vi "makeChangelogSVN.vi"(9 "end":string(combo) caption="endTagOrHash", 10 "start":string(combo) caption="startTagOrHash", 11 "VI Path":path) -> (1 "Changelog":string)   [LabVIEW 2022 SP3]
uses:
  d1585840-c92d-4c4b-9acf-e53ee60be502.vi
  <vilib>/Comparison/Less/Less Functor/Less Functor.lvclass
panel:
  in  "Tab Control":enum32{"changelog", "subVIs", "svn log"}(tab)
  out "subVIs":string[](array[string])
  out "standard output":string
  out "commandline":string="2.years"
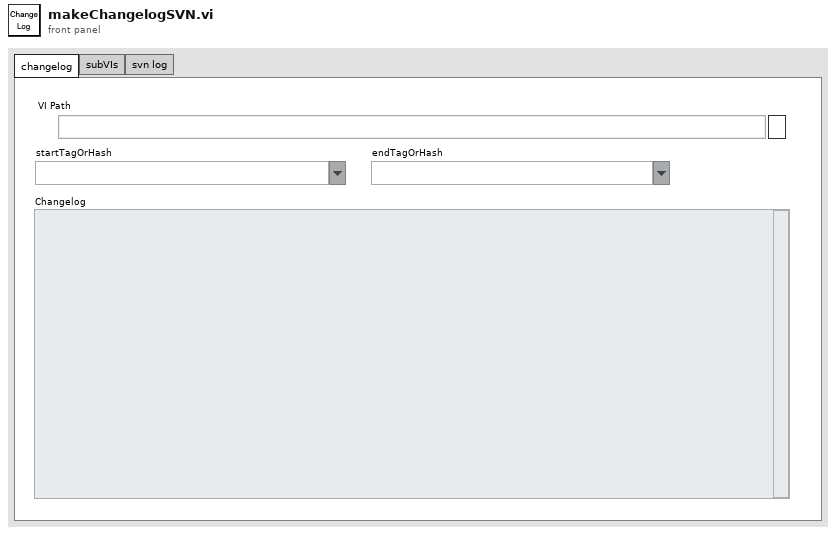
[diagram p1: front panel]
types:
  T1 = enum8{"Only include commented out diagrams if diagram already loaded", "Never include commented out diagrams", "Always include commented out diagrams"}
  T2 = enum8{"No dynamic dispatch VIs", "Include nearest implementation", "Include all overrides"}
  T3 = enum8{"Include the clone VI", "Include the original reentrant VI instead of the clone VI", "Include both the original reentrant VI and the clone VI"}
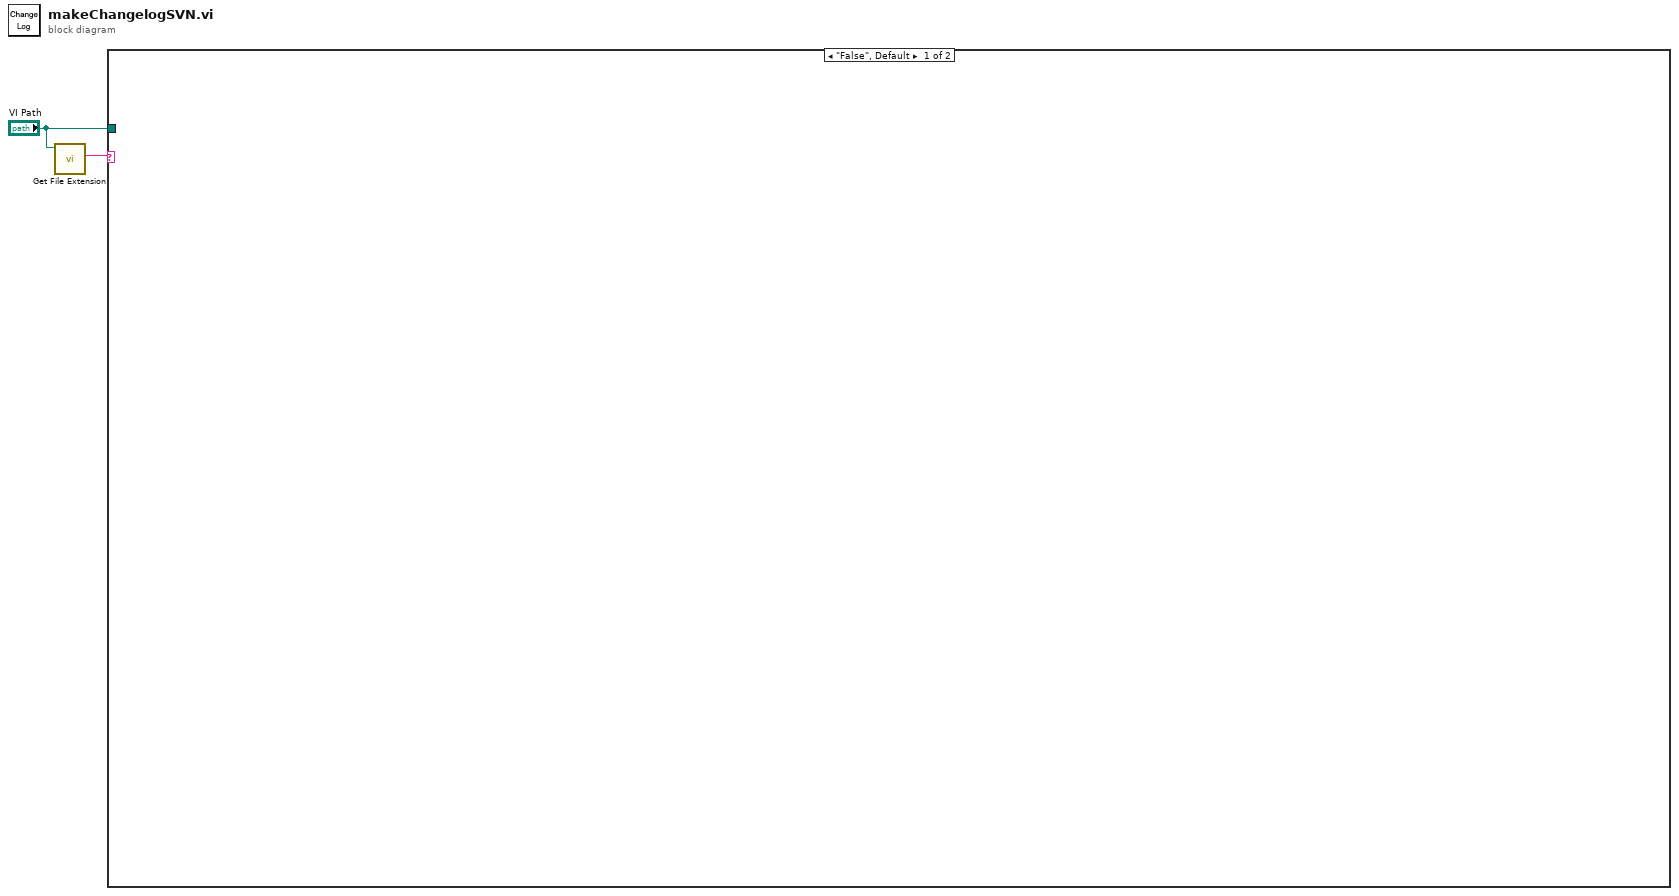
[diagram p0: block diagram]
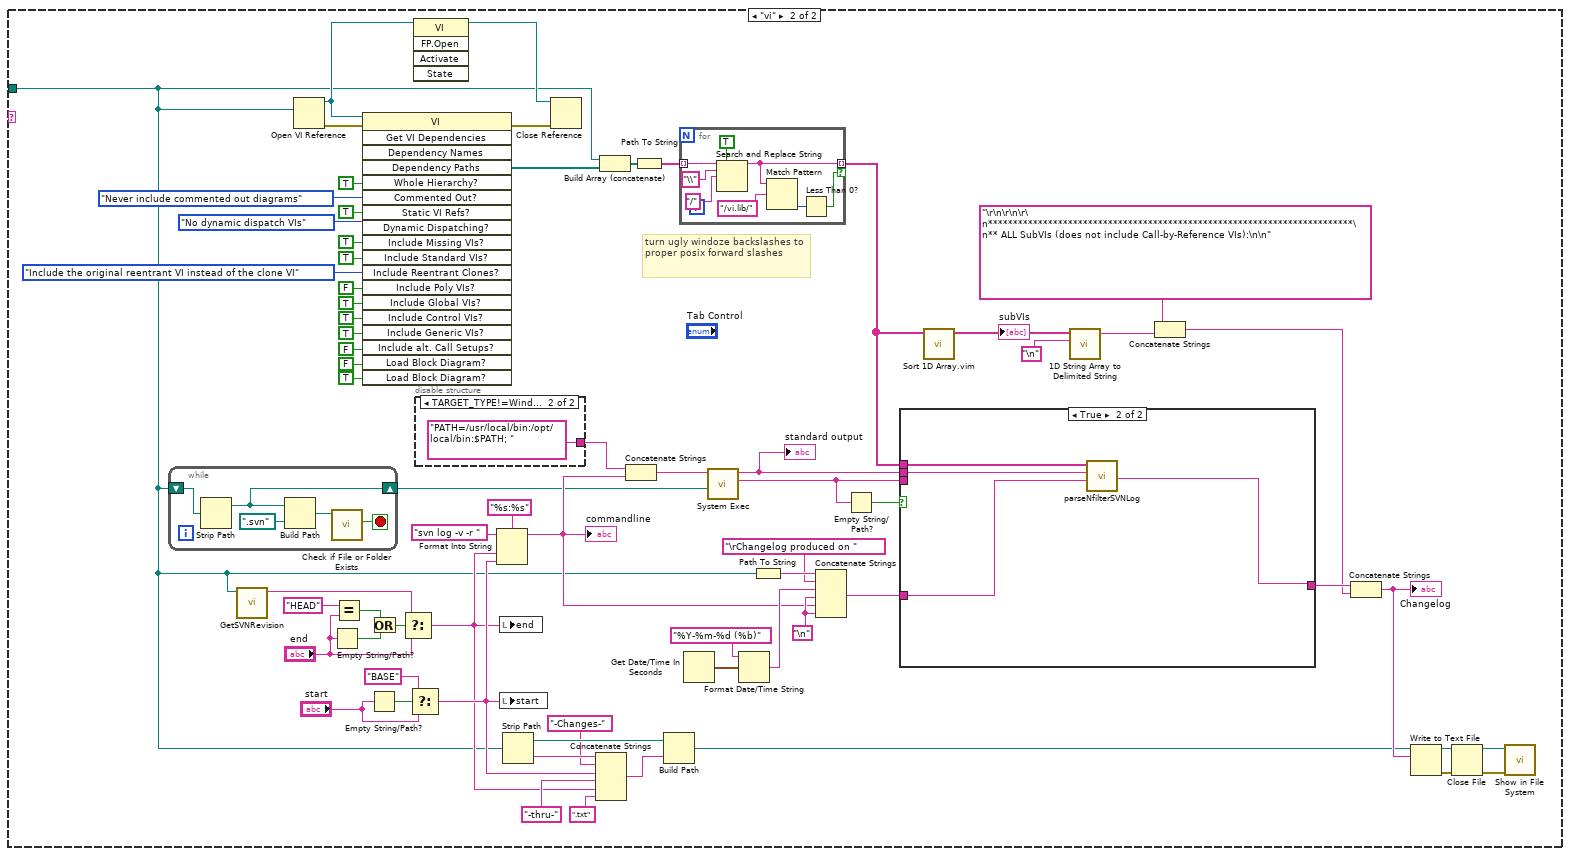
[diagram p2: hidden frame]
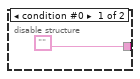
[diagram p3: hidden frame]
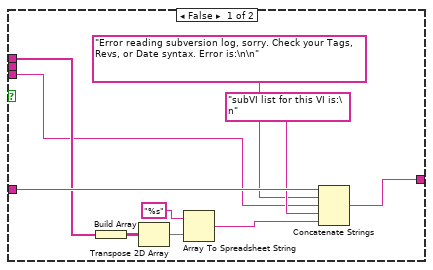
[diagram p4: hidden frame]
diagram:
  n1 = call <vilib>:"Get File Extension.vi"("file"="VI Path") -> ("lowercase file extension"=w2:string)  [unwired: 6 in, 4 out]
  n2 = case shown="\"False\", Default" w2 {
    tunnel: "VI Path" -> [_ w7]
    frame "False", Default {
    }
    frame "vi" {
      w50 = "\n"
      # "turn ugly windoze backslashes to proper posix forward slashes"
      n3 = while {
        shift-right: [w72] -> w10
        shift-left: w7 -> [w75]
        stop <- w71 stop-if-true
        n4 = Strip Path(path=w75) -> (stripped path=w72:path)  [unwired: 1 out]
        n5 = Build Path(base path=w72, name or relative path=path ".svn") -> (appended path=w73:path)
        n6 = call <vilib>:"Check if File or Folder Exists.vi"("path"=w73) -> ("file or folder exists?"=w71:bool)  [unwired: 8 in, 2 out]
      }
      n7 = call "GetSVNRevision.vi"("File Path Control"=w7) -> ("OverallRevision"=w8:string)  [unwired: 6 in, 4 out]
      n8 = Open VI Reference(vi path=w7) -> (vi reference=w11:refnum<vi>, error out=w59:errorcluster)  [unwired: 5 in]
      n9 = Empty String/Path?(string/path="end") -> (empty?=w17:bool)
      n10 = Equal?(x="HEAD", y="end") -> (x = y?=w3:bool)
      n11 = invoke class="VI" method="Get VI Dependencies"(reference=w11, error in=w59, "Whole Hierarchy?"=TRUE, "Commented Out?"=T1."Never include commented out diagrams" ("Commented Out Diagrams?"), "Static VI Refs?"=TRUE, "Dynamic Dispatching?"=T2."No dynamic dispatch VIs", "Include Missing VIs?"=TRUE ("Include Missing Items?"), "Include Standard VIs?"=TRUE, "Include Reentrant Clones?"=T3."Include the original reentrant VI instead of the clone VI", "Include Poly VIs?"=FALSE, "Include Global VIs?"=TRUE ("Include Control VIs?"), "Include Control VIs?"=TRUE, "Include Generic VIs?"=TRUE, "Include alt. Call Setups?"=FALSE ("Include Alternate Call Setups?"), "Load Block Diagram?"=FALSE ("Keep Express and Malleable VIs?"), "Load Block Diagram?"=TRUE) -> (error out=w61:errorcluster, "Dependency Paths"=w60:path[])  [unwired: 3 in, 17 out]
      n12 = Empty String/Path?(string/path="start") -> (empty?=w15:bool)
      n13 = Or(x=w3, y=w17) -> (x .or. y?=w4:bool)
      n14 = Select(t=w8, s=w4, f="end") -> (s? t:f=w12:string)
      n15 = Select(t="BASE", s=w15, f="start") -> (s? t:f=w13:string)
      n16 = invoke class="VI" method="FP.Open"(reference=w11) -> (reference out=w9:refnum<vi>)  [unwired: 4 in, 4 out]
      n17 = disable-structure shown="TARGET_TYPE!=Windows" {
        disable-tunnel: ["" ("command line") "PATH=/usr/local/bin:/opt/local/bin:$PATH; " ("command line")] -> w21
        frame condition #0 {
        }
        frame condition #1 (active) {
        }
      }
      n18 = Format Into String(format string="%s:%s", initial string="svn log -v -r " ("command line"), w12, w13) -> (resulting string=w18:string)  [unwired: 1 in, 1 out]
      "commandline" <- w18
      n19 = local write "end"(w12) -> ()
      n20 = local write "start"(w13) -> ()
      n21 = Strip Path(path=w7) -> (stripped path=w33:path, name=w32:string)
      n22 = Close Reference(reference=w9, error in (no error)=w61) -> ()  [unwired: 1 out]
      n23 = Concatenate Strings(w32, "-Changes-" ("string"), w13, "-thru-" ("string"), w12, ".txt" ("string")) -> (w31:string)
      n24 = Build Array (concatenate)(w7, w60) -> (w51:path[])
      n25 = Concatenate Strings(w21, w18) -> (w49:string)
      n26 = Path To String(path=w51) -> (string=w52:string[])
      n27 = Build Path(base path=w33, name or relative path=w31) -> (appended path=w30:path)
      n28 = for {
        tunnel: w52 -> [w85] mode=indexing
        tunnel: [w81] -> w48 mode=indexing if=w78
        n29 = Search and Replace String(replace all?=TRUE ("replace all? (F)"), input string=w85, search string="\\", replace string="/" ("replace string (\"\")")) -> (result string=w81:string)  [unwired: 4 in, 3 out]
        n30 = Match Pattern(string=w81, regular expression="/vi.lib/") -> (offset past match=w79:i32)  [unwired: 1 in, 3 out]
        n31 = Less Than 0?(x=w79) -> (x < 0?=w78:bool)
      }
      n32 = Get Date/Time In Seconds() -> (seconds since 1Jan1904=w66:timestamp)
      n33 = call <vilib>:"System Exec.vi"("working directory"=w10, "command line"=w49) -> ("standard error"=w22:string, "standard output"=w70:string)  [unwired: 6 in, 2 out]
      "standard output" <- w70
      n34 = Format Date/Time String(time format string (%c)="%Y-%m-%d (%b)", seconds (now)=w66) -> (date/time string=w67:string)  [unwired: 1 in]
      n35 = Path To String(path=w7) -> (string=w64:string)
      n36 = Concatenate Strings(w64, "\rChangelog produced on ", w67, w50, w18, w50) -> (w62:string)
      n37 = Empty String/Path?(string/path=w22) -> (empty?=w68:bool)
      n38 = case shown="True" w68 {
        tunnel: w70 -> [_ w98]
        tunnel: [w94 w96] -> w69
        tunnel: w62 -> [w95 w97]
        tunnel: w48 -> [w92 w99]
        tunnel: w22 -> [w86 _]
        frame False {
          n39 = Build Array(w92) -> (w90:string[][])
          n40 = Transpose 2D Array(2D array=w90) -> (transposed array=w89:string[][])
          n41 = Array To Spreadsheet String(array=w89, 3:"%s" ("format string")) -> (spreadsheet string=w93:string)  [unwired: 1 in]
          n42 = Concatenate Strings(w95, "Error reading subversion log, sorry. Check your Tags, Revs, or Date syntax. Error is:\n\n", w86, "subVI list for this VI is:\n" ("string"), w93) -> (w94:string)
        }
        frame True {
          n43 = call "parseNfilterSVNLog.vi"("changelogIn"=w97, "svnLog"=w98, "associatedVIs"=w99) -> ("relevantChangelogOut"=w96:string)  [unwired: 8 in]
        }
      }
      n44 = call "Sort 1D Array.vim"("unsorted array"=w48) -> ("sorted array"=w38:string[])  [unwired: 10 in]
      "subVIs" <- w38
      n45 = call <vilib>:"1D String Array to Delimited String.vi"("delimiter"="\n", "string array"=w38) -> ("delimited string"=w43:string)  [unwired: 9 in]
      n46 = Concatenate Strings("\r\n\r\n\r\n*************************************************************************\n** ALL SubVIs (does not include Call-by-Reference VIs):\n\n" ("string"), w43) -> (w41:string)
      n47 = Concatenate Strings(w69, w41) -> (w34:string)
      "Changelog" <- w34
      n48 = Write to Text File(file (use dialog)=w30, text=w34) -> (refnum out=w25:refnum<file>, error out=w26:errorcluster)  [unwired: 2 in, 1 out]
      n49 = Close File(refnum=w25, error in=w26) -> (path=w24:path, error out=w23:errorcluster)
      n50 = call <vilib>:"Show in File System.vi"("error in (no error)"=w23, "file or directory path"=w24) -> ()  [unwired: 9 in, 1 out]
    }
  }
